vi "Configure Trigger (Glitch).vi"(0 "VISA resource name":refnum<visa-resource-name>, 2 "Glitch Condition (0: Less Than)":u16(ring) items=["Less Than", "Greater Than"], 5 "Trigger Source (1: Channel 1)":u16(ring)=1 items=["Channel 1"=1, "Channel 2"=2, "Channel 3"=3, "Channel 4"=4, "External"=5, "External 5"=6], 7 "Glitch Polarity (0: Positive)":u16(ring) items=["Positive", "Negative"], 9 "Trigger Level (0.0 V)":dbl, 11 "error in (no error)":errorcluster, 12 "Glitch Width (1E-5 s)":dbl=1e-05, 13 "Trigger Modifier (0: Auto)":u16(ring) items=["Auto", "Normal", "Single"]) -> (4 "VISA resource name out":refnum<visa-resource-name>, 15 "error out":errorcluster)   [LabVIEW 2010, in "Agilent DSO1000 Series.lvlib"]
doc: "Configures the glitch trigger. A glitch trigger occurs when the trigger signal has a pulse with a width that is less than,greater than or equal to the glitch width based on the <B>Glitch Condition</B> control. You specify the glitch width in the <B>Glitch Width</B> control. You specify the polarity of the pulse with the <B>Glitch Polarity</B> control. The trigger does not actually occur until the edge of a pulse that corresponds to the <B>Glitch Width</B> value and <B>Glitch Polarity</B> value crosses the threshold you specify in the <B>Trigger Level</B> control."
uses:
  <instrlib>/Agilent DSO1000 Series/Agilent DSO1000 Series.lvlib
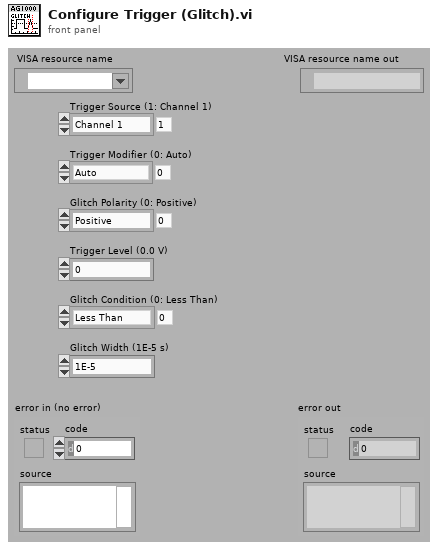
[diagram p1: front panel]
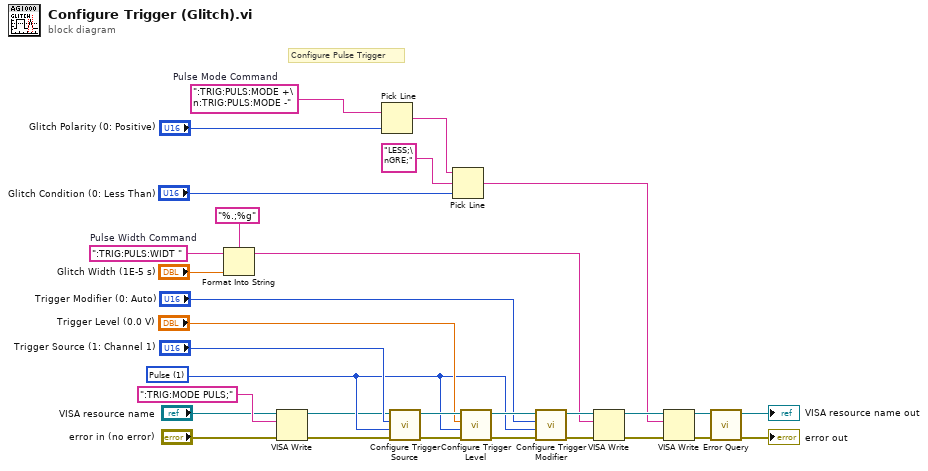
[diagram p0: block diagram]
diagram:
  w6 = u16 1 items=["Edge", "Pulse", "TV", "Pattern"] ("Trigger Type")
  w19 = ":TRIG:PULS:WIDT "  # Pulse Width Command
  w29 = ":TRIG:PULS:MODE +\n:TRIG:PULS:MODE -"  # Pulse Mode Command
  # "Configure Pulse Trigger"
  n1 = Format Into String(format string="%.;%g", initial string=w19, "Glitch Width (1E-5 s)") -> (resulting string=w15:string)  [unwired: 1 in, 1 out]
  n2 = VISA Write(VISA resource name="VISA resource name", write buffer=":TRIG:MODE PULS;", error in (no error)="error in (no error)") -> (VISA resource name out=w1:refnum<visa-resource-name>, error out=w3:errorcluster)  [unwired: 1 out]
  n3 = Pick Line(multi-line string=w29, line index="Glitch Polarity (0: Positive)") -> (output string=w12:string)  [unwired: 1 in]
  n4 = call <instrlib>:"Configure Trigger Source.vi"("error in (no error)"=w3, "Trigger Type"=w6, "Trigger Source (1: Channel 1)"="Trigger Source (1: Channel 1)", "VISA resource name"=w1) -> ("error out"=w26:errorcluster, "VISA resource name out"=w25:refnum<visa-resource-name>)  [unwired: 6 in]
  n5 = Pick Line(string ("")=w12, multi-line string="LESS;\nGRE;", line index="Glitch Condition (0: Less Than)") -> (output string=w7:string)
  n6 = call <instrlib>:"Configure Trigger Level.vi"("error in (no error)"=w26, "Trigger Type"=w6, "Trigger Level (0.0 V)"="Trigger Level (0.0 V)", "VISA resource name"=w25) -> ("error out"=w23:errorcluster, "VISA resource name out"=w22:refnum<visa-resource-name>)  [unwired: 6 in]
  n7 = call <instrlib>:"Configure Trigger Modifier.vi"("error in (no error)"=w23, "Trigger Type"=w6, "Trigger Modifier (0: Auto)"="Trigger Modifier (0: Auto)", "VISA resource name"=w22) -> ("error out"=w16:errorcluster, "VISA resource name out"=w17:refnum<visa-resource-name>)  [unwired: 6 in]
  n8 = VISA Write(VISA resource name=w17, write buffer=w15, error in (no error)=w16) -> (VISA resource name out=w10:refnum<visa-resource-name>, error out=w11:errorcluster)  [unwired: 1 out]
  n9 = VISA Write(VISA resource name=w10, write buffer=w7, error in (no error)=w11) -> (VISA resource name out=w9:refnum<visa-resource-name>, error out=w8:errorcluster)  [unwired: 1 out]
  n10 = call <instrlib>:"Error Query.vi"("error in (no error)"=w8, "VISA resource name"=w9) -> ("error out"=→"error out":errorcluster, "VISA resource name out"=→"VISA resource name out":refnum<visa-resource-name>)  [unwired: 6 in, 2 out]
